vi "TxBegin_Core.vi"(8 "error in (no error)":errorcluster, 11 "DbConnection in":refnum<class "DbConnection.lvclass">) -> (0 "error out":errorcluster, 3 "DbConnection out":refnum<class "DbConnection.lvclass">)   [LabVIEW 2020, in "ORM.lvlib" / "DbConnection.lvclass"]
uses:
  DbConnection.lvclass
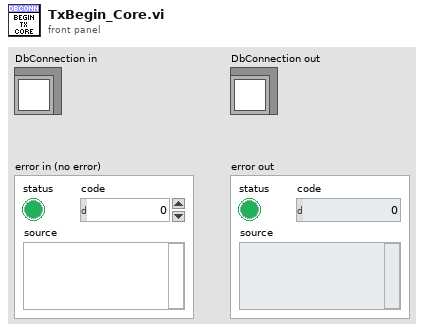
[diagram p1: front panel]
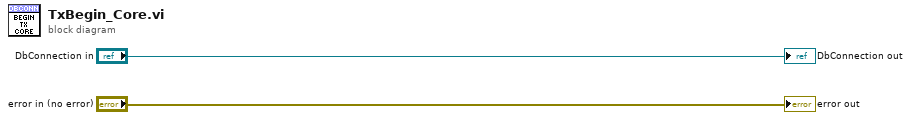
[diagram p0: block diagram]
diagram:
  "DbConnection out" <- "DbConnection in"
  "error out" <- "error in (no error)"
